vi "Pot Point.vi"(7 "Potting Surface Type":T1, 8 "error in":errorcluster, 10 "Point":refnum<class "Vec3d Class.lvclass">, 11 "SyringeTool in":refnum<class "SyringeTool Class.lvclass">) -> (0 "error out":errorcluster, 3 "SyringeTool out":refnum<class "SyringeTool Class.lvclass">)   [LabVIEW 2011, in "SyringeTool Class.lvclass"]
uses:
  SyringeTool Class.lvclass
  Vec3d Class/Vec3d Class.lvclass
  Config Manager Class/Type Definitions/Potting Surface Type.ctl
  WorkTable Class/WorkTable Class.lvclass
  Config Manager Class/Config Manager Class.lvclass
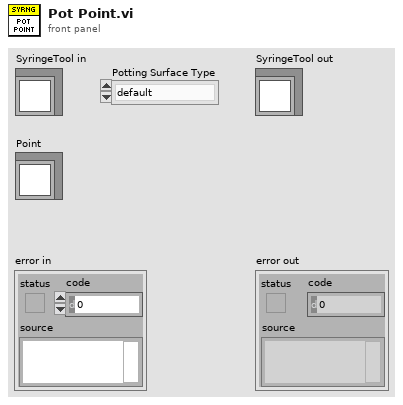
[diagram p1: front panel]
types:
  T1 = typedef "Potting Surface Type.ctl" = enum16{"default", "hdi_edge_pads"}
  T2 = typedef "Potting Parameters.ctl" = cluster{"Curing Param A":dbl, "Curing Param B":dbl, "Speed Nominal":dbl, "Time Nominal":dbl, "Turn-on Time":dbl, "Turn-off Time":dbl, "Safe Height Offset":dbl, "Tip Height":dbl, "Pot Length Scale":dbl}
  T3 = typedef "Worktable_Syringe.ctl" = cluster{"Syringe Holder":enum16{"Empty", "Populated", "Calibrated"}, "Mixing Time":timestamp, "Tip Offset":refnum<class "Vec3d Class.lvclass">}
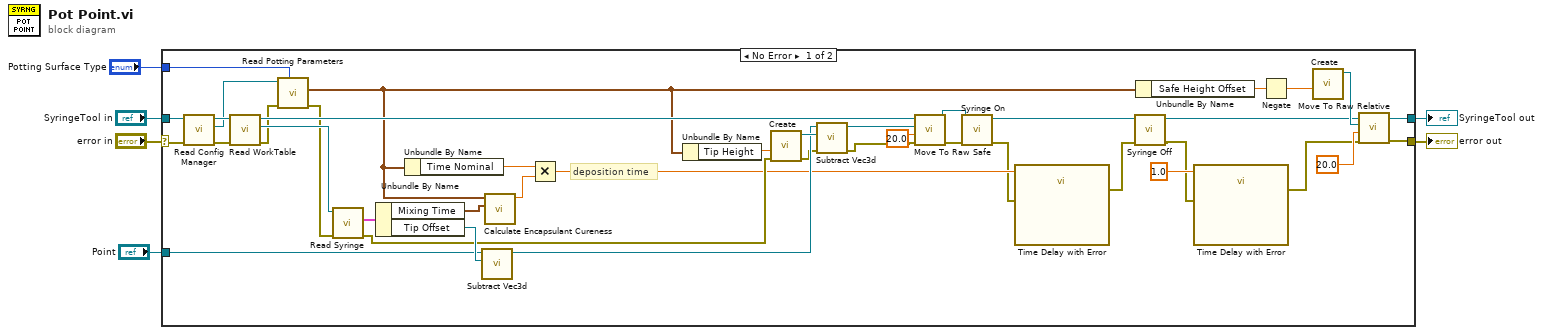
[diagram p0: block diagram]
diagram:
  n1 = case shown="No Error" "error in" {
    selector: "error in" -> [w30 w49]
    tunnel: [w44 w49] -> w3
    tunnel: [w45 w48] -> w4
    tunnel: "SyringeTool in" -> [w38 w48]
    tunnel: "Point" -> [w20 _]
    tunnel: "Potting Surface Type" -> [w13 _]
    frame No Error {
      # "deposition time"
      n2 = call-dynamic "Read Config Manager.vi"("error in"=w30, "Gantry in"=w38) -> ("error out"=w33:errorcluster, "Config Manager"=w34:refnum<class "Config Manager Class.lvclass">, "Gantry out"=w37:refnum<class "SyringeTool Class.lvclass">)  [unwired: 7 in]
      n3 = call-dynamic "Read WorkTable.vi"("error in"=w33, "Gantry Class in"=w37) -> ("error out"=w32:errorcluster, "WorkTable Class.lvclass"=w47:refnum<class "WorkTable Class.lvclass">, "Gantry Class out"=w43:refnum<class "SyringeTool Class.lvclass">)  [unwired: 7 in]
      n4 = call "Read Potting Parameters.vi"("Potting Surface Type"=w13, "error in"=w32, "Config Manager in"=w34) -> ("error out"=w31:errorcluster, "Potting Parameters"=w23:T2)  [unwired: 6 in, 1 out]
      n5 = call "Read Syringe.vi"("error in"=w31, "WorkTable in"=w47) -> ("error out"=w17:errorcluster, "Syringe"=w46:T3)  [unwired: 7 in, 1 out]
      n6 = Unbundle By Name(w46) -> ("Mixing Time"=w24:timestamp, "Tip Offset"=w42:refnum<class "Vec3d Class.lvclass">)
      n7 = Unbundle By Name(w23) -> ("Time Nominal"=w22:dbl)
      n8 = call "Subtract Vec3d.vi"("Vec3d in 2"=w42, "Vec3d in 1"=w20) -> ("Vec3d Class out"=w19:refnum<class "Vec3d Class.lvclass">)  [unwired: 8 in, 1 out]
      n9 = call "Calculate Encapsulant Cureness.vi"("Mixing Time"=w24, "Potting Parameters"=w23) -> ("Cureness"=w21:dbl)  [unwired: 8 in, 1 out]
      n10 = Multiply(x=w22, y=w21) -> (x*y=w9:dbl)
      n11 = Unbundle By Name(w23) -> ("Tip Height"=w27:dbl)
      n12 = call "Create.vi"("error in"=w17, "Z"=w27) -> ("error out"=w16:errorcluster, "Vec3d Class out"=w25:refnum<class "Vec3d Class.lvclass">)  [unwired: 8 in]
      n13 = call "Subtract Vec3d.vi"("error in (no error)"=w16, "Vec3d in 2"=w25, "Vec3d in 1"=w19) -> ("error out"=w15:errorcluster, "Vec3d Class out"=w26:refnum<class "Vec3d Class.lvclass">)  [unwired: 7 in]
      n14 = call-dynamic "Move To Raw Safe.vi"("error in"=w15, "Speed(mm/s)"=20.0, "Destination"=w26, "Gantry in"=w43) -> ("error out"=w41:errorcluster, "Gantry out"=w40:refnum<class "SyringeTool Class.lvclass">)  [unwired: 6 in]
      n15 = call "Syringe On.vi"("error in"=w41, "SyringeTool"=w40) -> ("error out"=w8:errorcluster, "SyringeTool out"=w18:refnum<class "SyringeTool Class.lvclass">)  [unwired: 8 in]
      n16 = call "Time Delay with Error.vi"("error in (no error)"=w8, "Delay Time (s)"=w9) -> ("error out"=w7:errorcluster)  [unwired: 9 in]
      n17 = call "Syringe Off.vi"("error in"=w7, "SyringeTool in"=w18) -> ("error out"=w11:errorcluster, "SyringeTool out"=w14:refnum<class "SyringeTool Class.lvclass">)  [unwired: 8 in]
      n18 = Unbundle By Name(w23) -> ("Safe Height Offset"=w36:dbl)
      n19 = call "Time Delay with Error.vi"("error in (no error)"=w11, "Delay Time (s)"=1.0) -> ("error out"=w10:errorcluster)  [unwired: 9 in]
      n20 = Negate(x=w36) -> (-x=w35:dbl)
      n21 = call "Create.vi"("Z"=w35) -> ("Vec3d Class out"=w39:refnum<class "Vec3d Class.lvclass">)  [unwired: 9 in, 1 out]
      n22 = call-dynamic "Move To Raw Relative.vi"("error in"=w10, "Speed(mm/s)"=20.0, "Delta"=w39, "Gantry in"=w14) -> ("error out"=w44:errorcluster, "Gantry out"=w45:refnum<class "SyringeTool Class.lvclass">)  [unwired: 6 in]
    }
    frame Error {
    }
  }
  "error out" <- w3
  "SyringeTool out" <- w4
